vi "AD7609 Get Nsamples Async.vi"() -> (1 "Channel volts":dbl[][](array[numeric]), 2 "Overruns":u32, 3 "Async error":errorcluster)   [LabVIEW 2015]
panel:
  # "PN 25/11/2014"
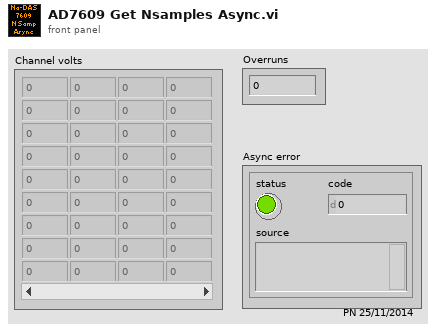
[diagram p1: front panel]
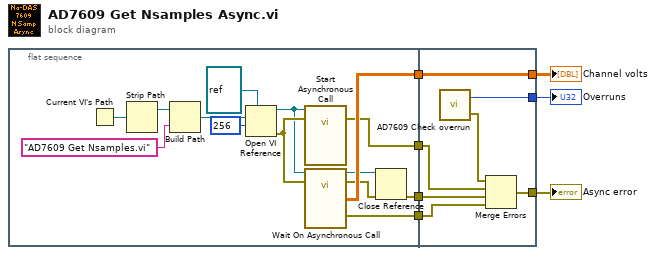
[diagram p0: block diagram]
diagram:
  n1 = flat-sequence {
    tunnel: [w18] -> w7
    tunnel: [w15] -> w4
    tunnel: [w10] -> w2
    tunnel: [w8] -> w1
    tunnel: [w28] -> w5
    tunnel: w7 -> [w28]
    tunnel: [w27] -> w6
    tunnel: [w22] -> w3
    tunnel: w4 -> [w25]
    tunnel: w2 -> [w26]
    tunnel: w1 -> [w24]
    frame #0 {
      n2 = Current VI's Path() -> (path=w14:path)
      n3 = Strip Path(path=w14) -> (stripped path=w13:path)  [unwired: 1 out]
      n4 = Build Path(base path=w13, name or relative path="AD7609 Get Nsamples.vi") -> (appended path=w11:path)
      n5 = Open VI Reference(type specifier VI Refnum (for type only)=refnum<vi> refnum, vi path=w11, options=256) -> (vi reference=w9:refnum<vi>, error out=w19:errorcluster)  [unwired: 3 in]
      n6 = call-by-ref "Start Asynchronous Call"(reference=w9, error in=w19) -> (error out=w10:errorcluster)  [unwired: 1 in, 3 out]
      n7 = call-by-ref "Wait On Asynchronous Call"(reference=w9, error in=w19) -> (reference out=w17:refnum<vi>, error out=w16:errorcluster, "Channel volts"=w18:dbl[][], 2:"error out"=w8:errorcluster)  [unwired: 1 in]
      n8 = Close Reference(reference=w17, error in (no error)=w16) -> (error out=w15:errorcluster)
    }
    frame #1 {
      n9 = call "AD7609 Check overrun.vi"() -> ("Overruns"=w27:u32, "Overrun error out"=w23:errorcluster)  [unwired: 1 in]
      n10 = Merge Errors(w23, w26, w25, w24) -> (w22:errorcluster)
    }
  }
  "Overruns" <- w6
  "Channel volts" <- w5
  "Async error" <- w3
